vi "WriteBinayFile.vi"   [LabVIEW 2020]
panel:
  # "Write  Binary File"
types:
  T1 = enum16{"open", "replace", "create", "open or create", "replace or create", "replace or create with confirmation"}
  T2 = enum16{"big-endian, network order", "native, host order", "little-endian"}
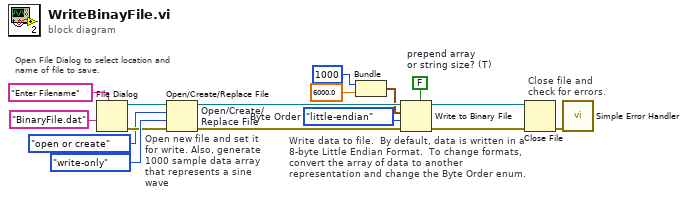
[diagram p0: block diagram]
diagram:
  w5 = T2."little-endian"  # Byte Order
  w6 = FALSE  # prepend array or string size? (T)
  # "Close file and check for errors."
  # "Write data to file.  By default, data is written in a 8-byte Little Endian Format.  To change formats, convert the array of data to another representation and change the Byte Order enum."
  # "Open new file and set it for write. Also, generate 1000 sample data array that represents a sine wave"
  # "Open File Dialog to select location and name of file to save."
  n1 = File Dialog(7:"Enter Filename" ("prompt"), 9:"BinaryFile.dat" ("default name")) -> (0:w7:errorcluster, 3:w16:path)  [unwired: 5 in, 2 out]
  n2 = Open/Create/Replace File "Open/Create/\nReplace File"(file path (use dialog)=w16, error in=w7, operation (0:open)=T1."open or create", access (0:read/write)=enum16{"read/write", "read-only", "write-only"}."write-only") -> (refnum out=w9:refnum<file>, error out=w10:errorcluster)  [unwired: 2 in, 1 out]
  n3 = Bundle("samples"=1000, "amplitude"=6000.0) -> (w1:cluster{"samples":i32, "amplitude":dbl})  [unwired: 1 in]
  n4 = Write to Binary File(file (use dialog)=w9, data=w1, error in=w10, 5:w6, 9:w5) -> (refnum out=w15:refnum<file>, error out=w13:errorcluster)  [unwired: 1 in, 1 out]
  n5 = Close File(refnum=w15, error in=w13) -> (error out=w12:errorcluster)  [unwired: 1 out]
  n6 = call <vilib>:"Simple Error Handler.vi"("error in (no error)"=w12) -> ()  [unwired: 4 in, 5 out]
